vi "Begin.vi"(8 "error in":errorcluster) -> (0 "error out":errorcluster)   [LabVIEW 2015]
doc: "Called before other user functions, this VI is expected to open initial I/O refnums, load in file data, and do all program initialization. Notice that the <B>error out</B> terminal is simply used for data flow. Wiring it to other structures or subVIs ensures that this VI runs first."
uses:
  <vilib>/Rock Robotics/WPI/DriverStation/WPI_DriverStationRobotMode2.ctl
  <vilib>/Rock Robotics/WPI/Joystick/WPI_JoystickDeviceEnum.ctl
  <vilib>/Rock Robotics/WPI/SafetyOutput/WPI_SafetyOutputConfigMenu.ctl
  <vilib>/Rock Robotics/SystemInterfaces/DIO/FPGA_DIOPWMChannel.ctl
  <vilib>/Rock Robotics/SystemInterfaces/AI/FPGA_AIGyroChannel.ctl
  <vilib>/Rock Robotics/SystemInterfaces/DIO/FPGA_DIOChannel.ctl
  <vilib>/Rock Robotics/WPI/Accelerometer/WPI_AccelerometerRange.ctl
  Robot Global Data.vi
  <vilib>/Rock Robotics/Network Tables/NT Write String Array.vi
  <vilib>/Rock Robotics/WPI/RobotDrive/WPI_RobotDriveOpen4MotorWithTalon.vi
  <vilib>/Rock Robotics/WPI/MotorControl/WPI_MotorControlOpen Talon.vi
  <vilib>/Rock Robotics/WPI/RobotDrive/WPI_RobotDriveOpen2MotorWithTalon.vi
  <vilib>/Rock Robotics/WPI/Accelerometer/InternalAccelerometer/WPI_AccelerometerInternalOpen.vi
  <vilib>/Rock Robotics/WPI/Counter/WPI_CounterDigitalInputToDigitalSource.vi
  <vilib>/Rock Robotics/WPI/Gyro/WPI_GyroAnalogOpen.vi
  <vilib>/Rock Robotics/WPI/MotorControl/WPI_MotorControlOpen Victor.vi
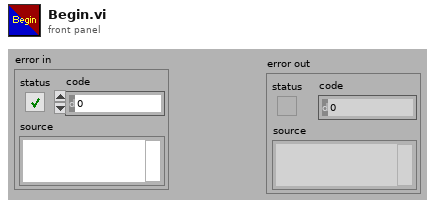
[diagram p1: front panel]
types:
  T1 = typedef "FPGA_DIOChannel.ctl" = enum8{"DIO 0", "DIO 1", "DIO 2", "DIO 3", "DIO 4", "DIO 5", "DIO 6", "DIO 7", "DIO 8", "DIO 9", "DIO MXP 0", "DIO MXP 1", "DIO MXP 2", "DIO MXP 3", "DIO MXP 4", "DIO MXP 5", "DIO MXP 6", "DIO MXP 7", "DIO MXP 8", "DIO MXP 9", "DIO MXP 10", "DIO MXP 11", "DIO MXP 12", "DIO MXP 13", "DIO MXP 14", "DIO MXP 15", "Invalid"}
  T2 = typedef "WPI_AccelerometerRange.ctl" = enum16{"+/- 2 g", "+/- 4 g", "+/- 8 g"}
  T3 = typedef "FPGA_AIGyroChannel.ctl" = enum8{"AI 0", "AI 1", "Invalid"}
  T4 = typedef "FPGA_DIOPWMChannel.ctl" = enum8{"PWM 0", "PWM 1", "PWM 2", "PWM 3", "PWM 4", "PWM 5", "PWM 6", "PWM 7", "PWM 8", "PWM 9", "PWM MXP 0", "PWM MXP 1", "PWM MXP 2", "PWM MXP 3", "PWM MXP 4", "PWM MXP 5", "PWM MXP 6", "PWM MXP 7", "PWM MXP 8", "PWM MXP 9", "Invalid"}
  T5 = typedef "WPI_JoystickDeviceEnum.ctl" = enum16{"USB 0", "USB 1", "USB 2", "USB 3", "USB 4", "USB 5"}
  T6 = typedef "WPI_SafetyOutputConfigMenu.ctl" = enum16{"Enable", "Disable"}
  T7 = typedef "WPI_DriverStationRobotMode2.ctl" = enum16{"Autonomous Disabled", "Autonomous Enabled", "Teleop Disabled", "Teleop Enabled", "Disconnected", "Finish", "Test Disabled", "Test Enabled", "Emergency Stopped"}
  T8 = typedef "WPI_MotorControlDeviceRef.ctl" = cluster{"DeviceStatus":errorcluster, "Type":T9, "PWM":cluster{"PWM Channel":T4, "DeadBand":T10}, "CAN":cluster{"Device Number":u8, "Control Mode":T11, "Semaphore":T12, "Max Vout":dbl, "TalonSRX Control Mode":T13}, "Invert":bool}
  T9 = typedef "WPI_MotorControlType.ctl" = enum16{"PWM", "CAN", "CANTalonSRX"}
  T10 = typedef "WPI_PWMDeadband.ctl" = cluster{"Name":string, "maxPositivePwm":i32, "minPositivePwm":i32, "centerPwm":i32, "maxNegativePwm":i32, "minNegativePwm":i32, "angularRange":u16}
  T11 = typedef "WPI_CANJaguar_ControlMode.ctl" = enum8{"Percent VBus", "Current", "Speed", "Position", "Voltage"}
  T12 = typedef "Semaphore RefNum" = refnum<k1>
  T13 = typedef "WPI_CANTalonSRX_APIControlMode.ctl" = enum8{"Percent VBus", "Speed", "Position", "Slave", "Unchanged / Invalid", "Voltage Compensation", "Current", "Motion Profile"}
  T14 = typedef "WPI_GyroDevRef.ctl" = cluster{"DevStatus":errorcluster, "Analog Channel":T15, "Offset":dbl, "Gain (VoltsPerDegree/Second)":dbl, "Gyro Type":enum16{"Analog", "XRS450"}, "Handle":i32, "SPI Bus":T16, "Device Found":bool, "Sample Rate":dbl, "Calibrate On Open":bool}
  T15 = typedef "FPGA_AIChannel.ctl" = enum8{"AI 0", "AI 1", "AI 2", "AI 3", "AI MXP 0", "AI MXP 1", "AI MXP 2", "AI MXP 3", "Invalid"}
  T16 = typedef "spi_bus.ctl" = enum16{"SPI On-Board, CS0", "SPI On-Board, CS1", "SPI On-Board, CS2", "SPI On-Board, CS3", "SPI MXP", "Invalid"}
  T17 = typedef "WPI_DigitalInputDevRef.ctl" = cluster{"DevStatus":errorcluster, "DIO Channel":T1}
  T18 = typedef "WPI_AccelerometerDevRef.ctl" = cluster{"DevStatus":errorcluster, "Scaling":T19, "Analog Channels":T20, "I2C Bus":T21, "SPI Bus":T16, "Accel Range":T22, "ADXL Axes":T23, "Handle":i32, "Device Address":u8, "Accel Type":enum16{"Analog", "ADXL345 I2C", "ADXL345 SPI", "Internal", "ADXL362 SPI"}}
  T19 = typedef "WPI_AccelerometerScaling.ctl" = cluster{"Gain (VoltsPerG)":dbl, "Center Voltage":dbl}
  T20 = typedef "WPI_AccelerometerAnalogChannels.ctl" = cluster{"X-Axis":T15, "Y-Axis":T15, "Z-Axis":T15}
  T21 = typedef "i2c_bus.ctl" = enum16{"I2C On-Board", "I2C MXP", "Invalid"}
  T22 = typedef "ADXL345 Range.ctl" = u8
  T23 = typedef "WPI_AccelerometerADXL345 Axes.ctl" = cluster{"X-Axis":bool, "Y-Axis":bool, "Z-Axis":bool}
  T24 = typedef "WPI_JoystickDevRef.ctl" = cluster{"Device":T5}
  T25 = typedef "WPI_RobotDriveDevRef.ctl" = cluster{"DevStatus":errorcluster, "Motors[]":T8[], "Square Inputs":bool, "Max Output":dbl}
  T26 = typedef "FPGA_CounterEncoderSourceConvertionLVSourceType.ctl" = cluster{"DevStatus":errorcluster, "AnalogTriggerMode?":bool, "DigitalMode":cluster{"DIO Channel":T27}, "AnalogTriggerMode":cluster{"AnalogTriggerIndex":T28, "OutputType":T29}}
  T27 = typedef "FPGA_DIODigitalSourceChannel.ctl" = enum8{"DIO 0", "DIO 1", "DIO 2", "DIO 3", "DIO 4", "DIO 5", "DIO 6", "DIO 7", "DIO 8", "DIO 9", "DIO MXP 0", "DIO MXP 1", "DIO MXP 2", "DIO MXP 3", "DIO MXP 4", "DIO MXP 5", "DIO MXP 6", "DIO MXP 7", "DIO MXP 8", "DIO MXP 9", "DIO MXP 10", "DIO MXP 11", "DIO MXP 12", "DIO MXP 13", "DIO MXP 14", "DIO MXP 15", "Disabled"}
  T28 = typedef "FPGA_AnalogTriggerIndex.ctl" = enum8{"Trig 0", "Trig 1", "Trig 2", "Trig 3", "Trig 4", "Trig 5", "Trig 6", "Trig 7", "Invalid"}
  T29 = typedef "FPGA_AnalogTriggerOutType.ctl" = enum16{"InWindow", "TriggerState", "Rising", "Falling"}
  T30 = typedef "WPI_EncoderDevRef.ctl" = cluster{"DevStatus":errorcluster, "EncoderIndex":T31, "CounterIndex":T32, "DistancePerCount":dbl, "Decoding Type":T33}
  T31 = typedef "FPGA_EncoderIdx.ctl" = enum8{"Enc 0", "Enc 1", "Enc 2", "Enc 3", "Enc 4", "Enc 5", "Enc 6", "Enc 7", "Invalid"}
  T32 = typedef "FPGA_CounterCtrSystemIndex.ctl" = enum8{"Ctr 0", "Ctr 1", "Ctr 2", "Ctr 3", "Ctr 4", "Ctr 5", "Ctr 6", "Ctr 7", "Invalid"}
  T33 = typedef "WPI_EncoderType.ctl" = enum16{"1x", "2x", "4x"}
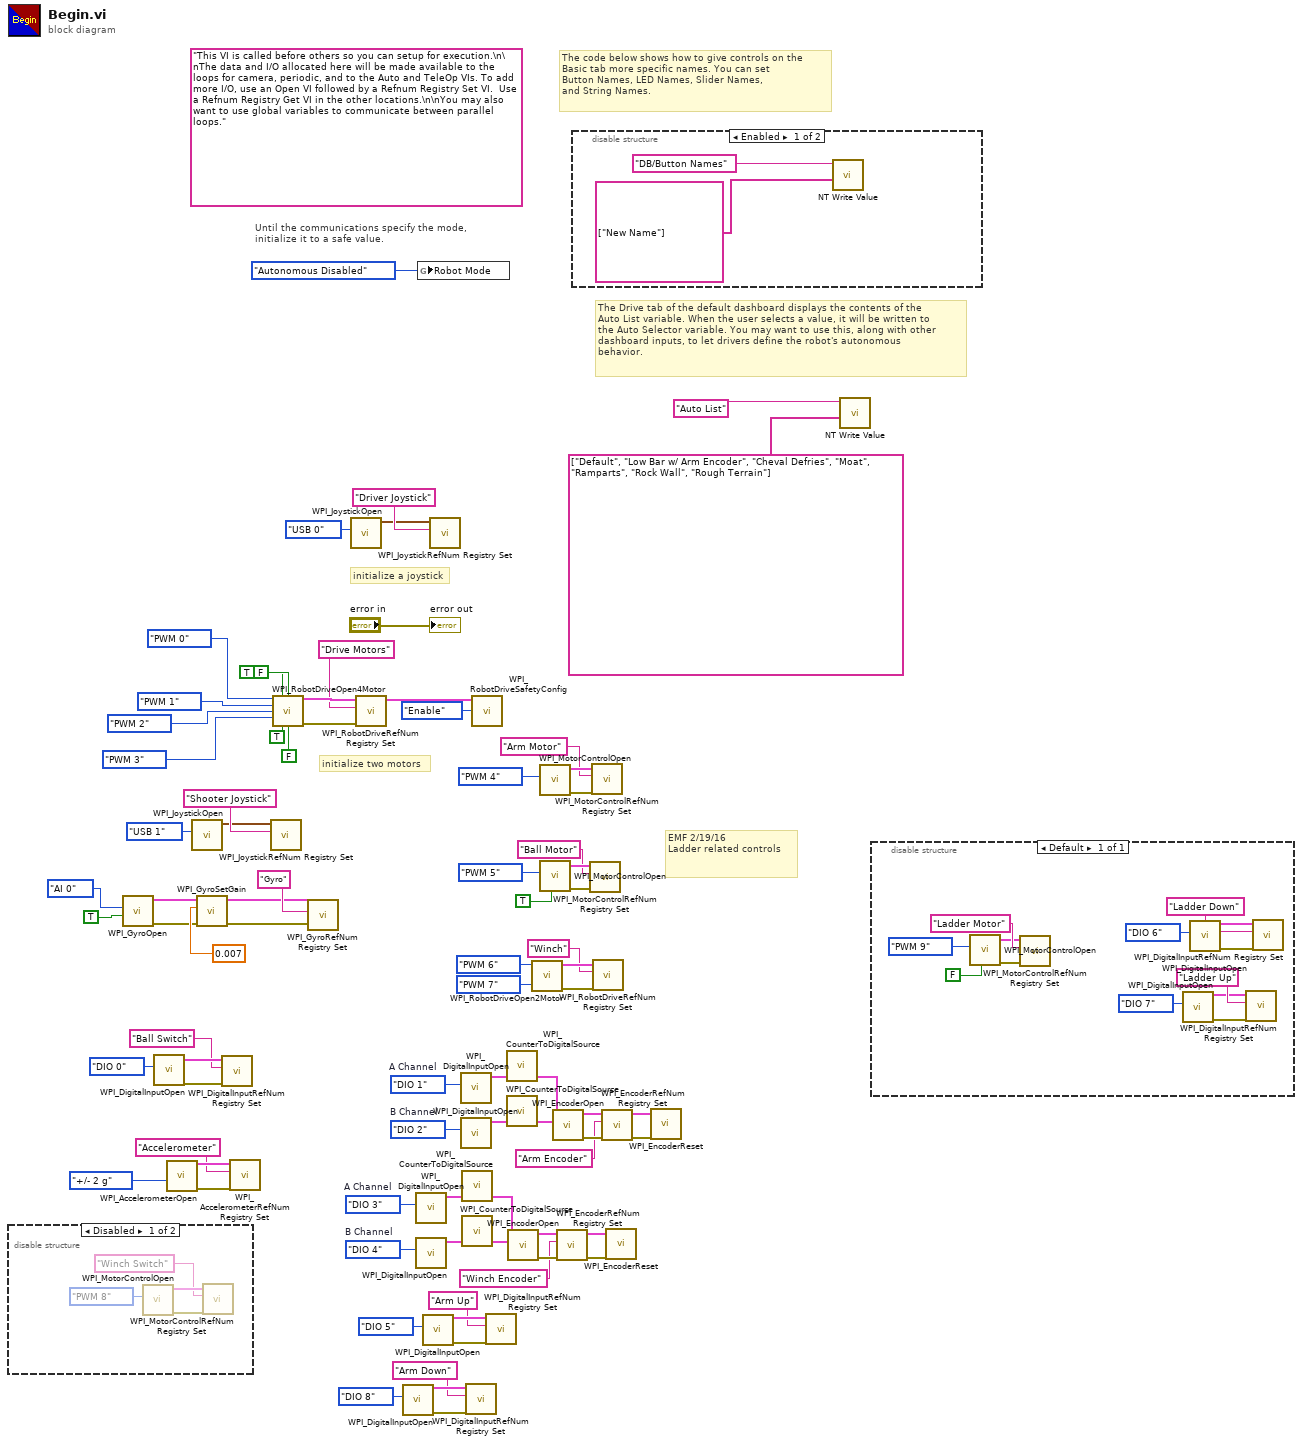
[diagram p0: block diagram]
diagram:
  w26 = FPGA_DIOChannel."DIO 4"  # B Channel
  w25 = FPGA_DIOChannel."DIO 3"  # A Channel
  w37 = FPGA_DIOChannel."DIO 2"  # B Channel
  w36 = FPGA_DIOChannel."DIO 1"  # A Channel
  (unwired) "This VI is called before others so you can setup for execution.\n\nThe data and I/O allocated here will be made available to the loops for camera, periodic, and to the Auto and TeleOp VIs. To add more I/O, use an Open VI followed by a Refnum Registry Set VI.  Use a Refnum Registry Get VI in the other locations.\n\nYou may also want to use global variables to communicate between parallel loops."
  # "EMF 2/19/16\nLadder related controls"
  # "initialize two motors"
  # "The Drive tab of the default dashboard displays the contents of the\nAuto List variable. When the user selects a value, it will be written to\nthe Auto Selector variable. You may want to use this, along with other\ndashboard inputs, to let drivers define the robot's autonomous\nbehavior."
  # "The code below shows how to give controls on the\nBasic tab more specific names. You can set\nButton Names, LED Names, Slider Names,\nand String Names."
  # "initialize a joystick"
  # "Until the communications specify the mode,\ninitialize it to a safe value."
  n1 = disable-structure shown="Disabled" {
    frame Disabled {
      n2 = call-poly <vilib>:"WPI_MotorControlOpen.vi"("PWM Channel"=FPGA_DIOPWMChannel."PWM 8") -> ("error out"=w86:errorcluster, "MotorControlDeviceRef"=w85:T8)  [unwired: 9 in]
      n3 = call <vilib>:"WPI_MotorControlRefNum Registry Set.vi"("error in (no error)"=w86, "refnum name"="Winch Switch", "MotorControlDevRef"=w85) -> ()  [unwired: 7 in, 2 out]
    }
    frame Enabled {
    }
  }
  n4 = call-poly <vilib>:"WPI_GyroOpen.vi"("Calibrate On Open"=TRUE, "Analog Channel"=FPGA_AIGyroChannel."AI 0") -> ("error out"=w8:errorcluster, "GyroDevRef"=w11:T14)  [unwired: 7 in, 1 out]
  n5 = call <vilib>:"WPI_DigitalInputOpen.vi"("DIO Channel"=FPGA_DIOChannel."DIO 0") -> ("error out"=w42:errorcluster, "DigitalInputDevRef"=w44:T17)  [unwired: 9 in]
  n6 = call-poly <vilib>:"WPI_AccelerometerOpen.vi"("Accel Range"=WPI_AccelerometerRange."+/- 2 g") -> ("error out"=w39:errorcluster, "AccelerometerDevRef"=w40:T18)  [unwired: 9 in]
  n7 = call <vilib>:"WPI_JoystickOpen.vi"("JoystickDevice"=WPI_JoystickDeviceEnum."USB 1") -> ("JoystickDevRef"=w62:T24)  [unwired: 10 in]
  n8 = call <vilib>:"WPI_GyroSetGain.vi"("error in (no error)"=w8, "Gain (VoltsPerDegree/Second)"=0.007, "GyroDevRef"=w11) -> ("error out"=w6:errorcluster, "GyroDevRef"=w9:T14)  [unwired: 7 out]
  n9 = call <vilib>:"WPI_DigitalInputRefNum Registry Set.vi"("error in (no error)"=w42, "refnum name"="Ball Switch", "DigitalInputDevRef"=w44) -> ()  [unwired: 7 in, 2 out]
  n10 = call <vilib>:"WPI_AccelerometerRefNum Registry Set.vi"("error in (no error)"=w39, "refnum name"="Accelerometer", "AccelerometerDevRef"=w40) -> ()  [unwired: 7 in, 2 out]
  n11 = call <vilib>:"WPI_JoystickRefNum Registry Set.vi"("refnum name"="Shooter Joystick", "JoystickDevRef"=w62) -> ()  [unwired: 8 in, 2 out]
  n12 = call-poly <vilib>:"WPI_RobotDriveOpen4Motor.vi"("Rear Left Motor"=FPGA_DIOPWMChannel."PWM 0", "Rear Left Motor Inverted"=TRUE, "Rear Right Motor Inverted"=FALSE, "Rear Right Motor"=FPGA_DIOPWMChannel."PWM 1", "Front Left Motor"=FPGA_DIOPWMChannel."PWM 2", "Front Right Motor"=FPGA_DIOPWMChannel."PWM 3", "Front Left Motor Inverted"=TRUE, "Front Right Motor Inverted"=FALSE) -> ("RobotDriveDevRef"=w76:T25, "error out"=w74:errorcluster)  [unwired: 6 in]
  n13 = call <vilib>:"WPI_GyroRefNum Registry Set.vi"("error in (no error)"=w6, "refnum name"="Gyro", "GyroDevRef"=w9) -> ()  [unwired: 7 in, 2 out]
  n14 = call <vilib>:"WPI_JoystickOpen.vi"("JoystickDevice"=WPI_JoystickDeviceEnum."USB 0") -> ("JoystickDevRef"=w81:T24)  [unwired: 10 in]
  n15 = call <vilib>:"WPI_RobotDriveRefNum Registry Set.vi"("error in (no error)"=w74, "refnum name"="Drive Motors", "RobotDriveDevRef"=w76) -> ("RobotDriveDevRef"=w73:T25)  [unwired: 1 in, 7 out]
  n16 = call <vilib>:"WPI_DigitalInputOpen.vi"("DIO Channel"=FPGA_DIOChannel."DIO 8") -> ("error out"=w3:errorcluster, "DigitalInputDevRef"=w4:T17)  [unwired: 9 in]
  n17 = call <vilib>:"WPI_DigitalInputOpen.vi"("DIO Channel"=w25) -> ("DigitalInputDevRef"=w22:T17)  [unwired: 1 in, 9 out]
  n18 = call <vilib>:"WPI_DigitalInputOpen.vi"("DIO Channel"=w26) -> ("DigitalInputDevRef"=w23:T17)  [unwired: 1 in, 9 out]
  n19 = global write "Robot Global Data.vi" "Robot Mode"(WPI_DriverStationRobotMode2."Autonomous Disabled" ("Robot Mode")) -> ()
  n20 = call <vilib>:"WPI_DigitalInputOpen.vi"("DIO Channel"=FPGA_DIOChannel."DIO 5") -> ("error out"=w13:errorcluster, "DigitalInputDevRef"=w14:T17)  [unwired: 9 in]
  n21 = call <vilib>:"WPI_JoystickRefNum Registry Set.vi"("refnum name"="Driver Joystick", "JoystickDevRef"=w81) -> ()  [unwired: 8 in, 2 out]
  n22 = call <vilib>:"WPI_DigitalInputOpen.vi"("DIO Channel"=w36) -> ("DigitalInputDevRef"=w33:T17)  [unwired: 1 in, 9 out]
  n23 = call <vilib>:"WPI_DigitalInputOpen.vi"("DIO Channel"=w37) -> ("DigitalInputDevRef"=w34:T17)  [unwired: 1 in, 9 out]
  n24 = call-poly <vilib>:"WPI_CounterToDigitalSource.vi"("DigitalInputDevRef"=w22) -> ("Digital Source"=w21:T26)  [unwired: 6 out]
  n25 = call-poly <vilib>:"WPI_CounterToDigitalSource.vi"("DigitalInputDevRef"=w23) -> ("Digital Source"=w24:T26)  [unwired: 6 out]
  n26 = call <vilib>:"WPI_DigitalInputRefNum Registry Set.vi"("error in (no error)"=w3, "refnum name"="Arm Down", "DigitalInputDevRef"=w4) -> ()  [unwired: 7 in, 2 out]
  n27 = call <vilib>:"WPI_RobotDriveSafetyConfig.vi"("mode"=WPI_SafetyOutputConfigMenu."Enable", "RobotDriveDevRef"=w73) -> ()  [unwired: 8 in, 2 out]
  n28 = call <vilib>:"WPI_DigitalInputRefNum Registry Set.vi"("error in (no error)"=w13, "refnum name"="Arm Up", "DigitalInputDevRef"=w14) -> ()  [unwired: 7 in, 2 out]
  n29 = call-poly <vilib>:"WPI_CounterToDigitalSource.vi"("DigitalInputDevRef"=w33) -> ("Digital Source"=w32:T26)  [unwired: 6 out]
  n30 = call-poly <vilib>:"WPI_CounterToDigitalSource.vi"("DigitalInputDevRef"=w34) -> ("Digital Source"=w35:T26)  [unwired: 6 out]
  n31 = call <vilib>:"WPI_EncoderOpen.vi"("BSource"=w24, "ASource"=w21) -> ("error out"=w20:errorcluster, "EncoderDevRef"=w19:T30)  [unwired: 6 in, 2 out]
  n32 = call-poly <vilib>:"WPI_RobotDriveOpen2Motor.vi"("Right Motor"=FPGA_DIOPWMChannel."PWM 7", "Left Motor"=FPGA_DIOPWMChannel."PWM 6") -> ("error out"=w47:errorcluster, "RobotDriveDevRef"=w49:T25)  [unwired: 8 in]
  n33 = call-poly <vilib>:"WPI_MotorControlOpen.vi"("PWM Channel"=FPGA_DIOPWMChannel."PWM 4") -> ("error out"=w58:errorcluster, "MotorControlDeviceRef"=w57:T8)  [unwired: 9 in]
  n34 = call-poly <vilib>:"WPI_MotorControlOpen.vi"("Invert"=TRUE, "PWM Channel"=FPGA_DIOPWMChannel."PWM 5") -> ("error out"=w54:errorcluster, "MotorControlDeviceRef"=w55:T8)  [unwired: 8 in]
  n35 = call <vilib>:"WPI_EncoderOpen.vi"("BSource"=w35, "ASource"=w32) -> ("error out"=w31:errorcluster, "EncoderDevRef"=w30:T30)  [unwired: 6 in, 2 out]
  n36 = call <vilib>:"WPI_EncoderRefNum Registry Set.vi"("error in (no error)"=w20, "refnum name"="Winch Encoder", "EncoderDevRef"=w19) -> ("error out"=w17:errorcluster, "EncoderDevRef"=w16:T30)  [unwired: 7 in]
  n37 = disable-structure shown="Enabled" {
    frame Enabled {
      n38 = call-poly <vilib>:"NT Write Value.vi"("String Array"=string[] ["New Name"], "Name"="DB/Button Names") -> ()  [unwired: 9 in, 1 out]
    }
    frame Disabled {
    }
  }
  n39 = call <vilib>:"WPI_MotorControlRefNum Registry Set.vi"("error in (no error)"=w54, "refnum name"="Ball Motor", "MotorControlDevRef"=w55) -> ()  [unwired: 7 in, 2 out]
  n40 = call <vilib>:"WPI_MotorControlRefNum Registry Set.vi"("error in (no error)"=w58, "refnum name"="Arm Motor", "MotorControlDevRef"=w57) -> ()  [unwired: 7 in, 2 out]
  n41 = call <vilib>:"WPI_RobotDriveRefNum Registry Set.vi"("error in (no error)"=w47, "refnum name"="Winch", "RobotDriveDevRef"=w49) -> ()  [unwired: 7 in, 2 out]
  n42 = call <vilib>:"WPI_EncoderRefNum Registry Set.vi"("error in (no error)"=w31, "refnum name"="Arm Encoder", "EncoderDevRef"=w30) -> ("error out"=w28:errorcluster, "EncoderDevRef"=w27:T30)  [unwired: 7 in]
  n43 = call <vilib>:"WPI_EncoderReset.vi"("error in (no error)"=w17, "EncoderDevRef"=w16) -> ()  [unwired: 8 in, 2 out]
  n44 = call <vilib>:"WPI_EncoderReset.vi"("error in (no error)"=w28, "EncoderDevRef"=w27) -> ()  [unwired: 8 in, 2 out]
  n45 = call-poly <vilib>:"NT Write Value.vi"("String Array"=string[] ["Default", "Low Bar w/ Arm Encoder", "Cheval Defries", "Moat", "Ramparts", "Rock Wall", "Rough Terrain"], "Name"="Auto List") -> ()  [unwired: 9 in, 1 out]
  n46 = disable-structure shown="Default" {
    frame Enabled {
      n47 = call-poly <vilib>:"WPI_MotorControlOpen.vi"("Invert"=FALSE, "PWM Channel"=FPGA_DIOPWMChannel."PWM 9") -> ("error out"=w92:errorcluster, "MotorControlDeviceRef"=w91:T8)  [unwired: 8 in]
      n48 = call <vilib>:"WPI_MotorControlRefNum Registry Set.vi"("error in (no error)"=w92, "refnum name"="Ladder Motor", "MotorControlDevRef"=w91) -> ()  [unwired: 7 in, 2 out]
      n49 = call <vilib>:"WPI_DigitalInputOpen.vi"("DIO Channel"=FPGA_DIOChannel."DIO 7") -> ("error out"=w101:errorcluster, "DigitalInputDevRef"=w100:T17)  [unwired: 9 in]
      n50 = call <vilib>:"WPI_DigitalInputOpen.vi"("DIO Channel"=FPGA_DIOChannel."DIO 6") -> ("error out"=w97:errorcluster, "DigitalInputDevRef"=w96:T17)  [unwired: 9 in]
      n51 = call <vilib>:"WPI_DigitalInputRefNum Registry Set.vi"("error in (no error)"=w101, "refnum name"="Ladder Up", "DigitalInputDevRef"=w100) -> ()  [unwired: 7 in, 2 out]
      n52 = call <vilib>:"WPI_DigitalInputRefNum Registry Set.vi"("error in (no error)"=w97, "refnum name"="Ladder Down", "DigitalInputDevRef"=w96) -> ()  [unwired: 7 in, 2 out]
    }
  }
  "error out" <- "error in"
